vi "Digital Input Data.vi"(8 "error in (no error)":errorcluster, 10 "Digital Data":bool[](array[boolean]), 11 "Root Tester in":refnum<class "Root Tester.lvclass">) -> (0 "error out":errorcluster, 3 "Root Tester out":refnum<class "Root Tester.lvclass">)   [LabVIEW 2024, in "Root Tester.lvlib" / "Root Tester.lvclass"]
uses:
  Root Tester.lvclass
  Root Tester.lvclass/Root Tester.ctl
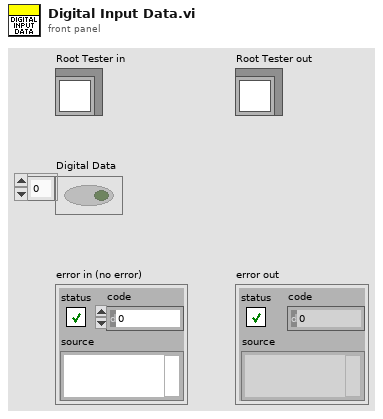
[diagram p1: front panel]
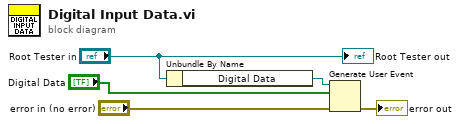
[diagram p0: block diagram]
diagram:
  n1 = Unbundle By Name("Root Tester in") -> ("Digital Data"=w4:refnum<user-event>)
  n2 = Generate User Event(user event=w4, event data cluster="Digital Data", error in="error in (no error)") -> (error out=→"error out":errorcluster)  [unwired: 1 in, 1 out]
  "Root Tester out" <- "Root Tester in"
